vi "peak_value_calculate_A_4_zero_negatives.vi"(0 "IO Module\\AI 1 Data N-1 2":i16, 1 "IO Module\\AI 1 Data N-2 3":i16, 2 "IO Module\\AI 1 Data N-2 2":i16, 3 "Boolean in":bool, 4 "IO Module\\AI 1 Data N-3 2":i16, 6 "IO Module\\AI 1 Data N 3":i16, 7 "IO Module\\AI 1 Data N":i16, 8 "IO Module\\AI 1 Data N-1 3":i16, 9 "IO Module\\AI 1 Data N-3":i16, 10 "IO Module\\AI 1 Data N 2":i16, 11 "IO Module\\AI 1 Data N-1":i16, 13 "IO Module\\AI 1 Data N-2":i16) -> (15 "Read Ready":bool, 16 "Spike Value":i16)   [LabVIEW 2017]
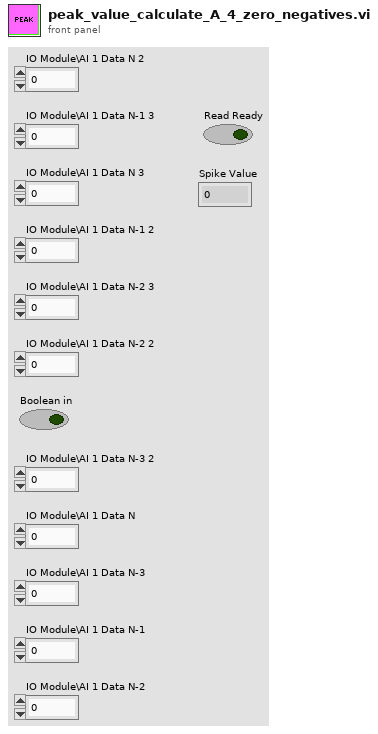
[diagram p1: front panel]
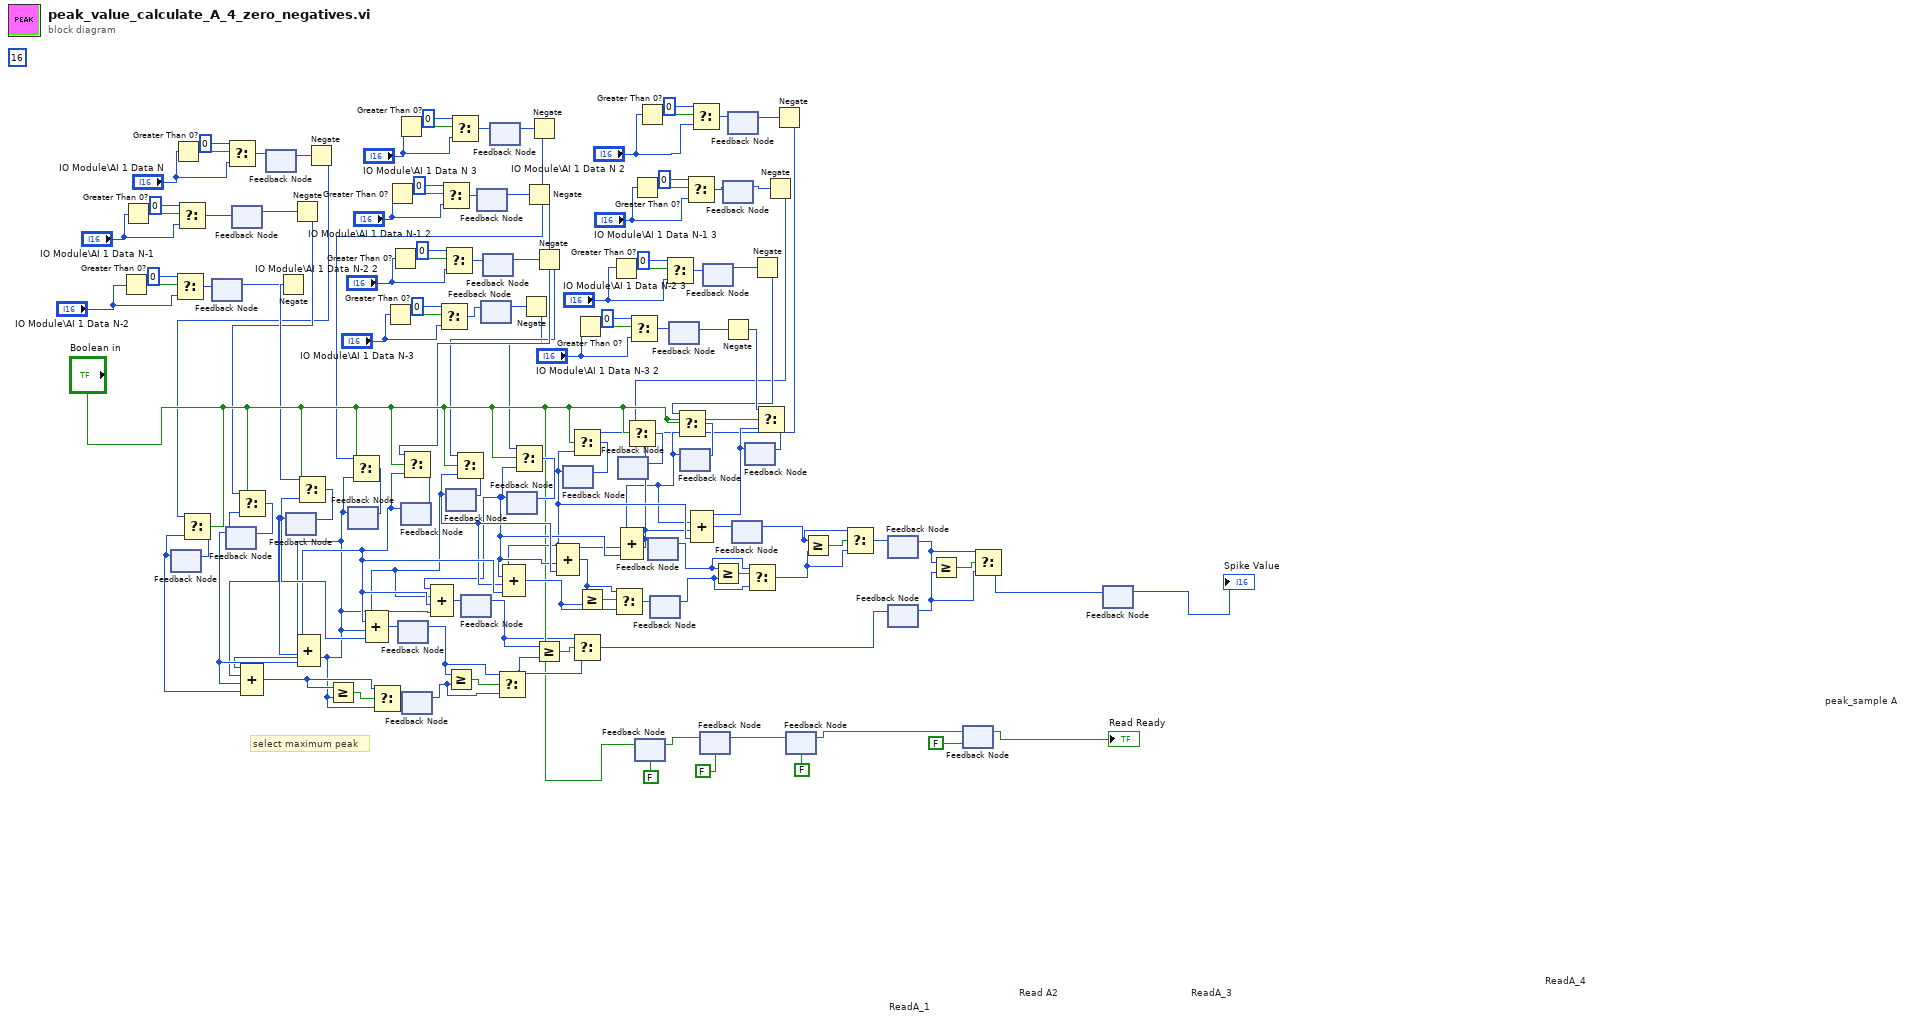
[diagram p0: block diagram]
diagram:
  (unwired) 16
  # "select maximum peak"
  n1 = Greater Than 0?(x="IO Module\\AI 1 Data N-2") -> (x > 0?=w43:bool)
  n2 = Greater Than 0?(x="IO Module\\AI 1 Data N-1") -> (x > 0?=w46:bool)
  n3 = feedback #1() -> (w110:i16)  [unwired: 1 in]
  n4 = Greater Than 0?(x="IO Module\\AI 1 Data N") -> (x > 0?=w49:bool)
  n5 = Select(t=i16 0, s=w43, f="IO Module\\AI 1 Data N-2") -> (s? t:f=w41:i16)
  n6 = Select(t=i16 0, s=w46, f="IO Module\\AI 1 Data N-1") -> (s? t:f=w44:i16)
  n7 = feedback-in #2(w41) -> ()
  n8 = feedback #2() -> (w9:i16)  [unwired: 1 in]
  n9 = feedback #3() -> (w109:i16)  [unwired: 1 in]
  n10 = Select(t=i16 0, s=w49, f="IO Module\\AI 1 Data N") -> (s? t:f=w47:i16)
  n11 = feedback-in #4(w44) -> ()
  n12 = feedback #4() -> (w10:i16)  [unwired: 1 in]
  n13 = feedback-in #5(w47) -> ()
  n14 = feedback #5() -> (w11:i16)  [unwired: 1 in]
  n15 = Negate(x=w9) -> (-x=w22:i16)
  n16 = feedback #6() -> (w106:i16)  [unwired: 1 in]
  n17 = Negate(x=w10) -> (-x=w21:i16)
  n18 = Select(t=w21, s="Boolean in", f=w109) -> (s? t:f=w114:i16)
  n19 = feedback-in #3(w114) -> ()
  n20 = Select(t=w22, s="Boolean in", f=w106) -> (s? t:f=w115:i16)
  n21 = feedback-in #6(w115) -> ()
  n22 = Negate(x=w11) -> (-x=w20:i16)
  n23 = Select(t=w20, s="Boolean in", f=w110) -> (s? t:f=w120:i16)
  n24 = feedback-in #1(w120) -> ()
  n25 = feedback #7() -> (w96:i16)  [unwired: 1 in]
  n26 = Compound Arithmetic op=ADD(w96, w106, w109, w110) -> (w97:i16)
  n27 = Greater Or Equal?(x=w97, y=w96) -> (x >= y?=w98:bool)
  n28 = Select(t=w97, s=w98, f=w96) -> (s? t:f=w122:i16)
  n29 = Greater Than 0?(x="IO Module\\AI 1 Data N-3") -> (x > 0?=w52:bool)
  n30 = Greater Than 0?(x="IO Module\\AI 1 Data N-1 2") -> (x > 0?=w58:bool)
  n31 = Greater Than 0?(x="IO Module\\AI 1 Data N-2 2") -> (x > 0?=w55:bool)
  n32 = Greater Than 0?(x="IO Module\\AI 1 Data N 3") -> (x > 0?=w61:bool)
  n33 = feedback #8() -> (w18:i16)  [unwired: 1 in]
  n34 = feedback #9() -> (w105:i16)  [unwired: 1 in]
  n35 = Compound Arithmetic op=ADD(w105, w96, w106, w109) -> ()  [unwired: 1 out]
  n36 = feedback-in #10(w122) -> ()
  n37 = feedback #10() -> (w19:i16)  [unwired: 1 in]
  n38 = Select(t=i16 0, s=w52, f="IO Module\\AI 1 Data N-3") -> (s? t:f=w50:i16)
  n39 = Select(t=i16 0, s=w58, f="IO Module\\AI 1 Data N-1 2") -> (s? t:f=w56:i16)
  n40 = Select(t=i16 0, s=w55, f="IO Module\\AI 1 Data N-2 2") -> (s? t:f=w53:i16)
  n41 = feedback #11() -> (w104:i16)  [unwired: 1 in]
  n42 = Compound Arithmetic op=ADD(w104, w105, w96, w106) -> (w95:i16)
  n43 = feedback-in #8(w95) -> ()
  n44 = Greater Or Equal?(x=w18, y=w19) -> (x >= y?=w123:bool)
  n45 = Select(t=i16 0, s=w61, f="IO Module\\AI 1 Data N 3") -> (s? t:f=w59:i16)
  n46 = feedback #12() -> (w17:i16)  [unwired: 1 in]
  n47 = feedback-in #13(w56) -> ()
  n48 = feedback #13() -> (w7:i16)  [unwired: 1 in]
  n49 = feedback-in #14(w50) -> ()
  n50 = feedback #14() -> (w5:i16)  [unwired: 1 in]
  n51 = feedback-in #15(w53) -> ()
  n52 = feedback #15() -> (w6:i16)  [unwired: 1 in]
  n53 = feedback-in #16(w59) -> ()
  n54 = feedback #16() -> (w8:i16)  [unwired: 1 in]
  n55 = Select(t=w18, s=w123, f=w19) -> (s? t:f=w92:i16)
  n56 = feedback #17() -> (w103:i16)  [unwired: 1 in]
  n57 = Compound Arithmetic op=ADD(w103, w104, w105, w96) -> (w93:i16)
  n58 = feedback-in #12(w93) -> ()
  n59 = Negate(x=w5) -> (-x=w23:i16)
  n60 = Select(t=w23, s="Boolean in", f=w103) -> (s? t:f=w119:i16)
  n61 = feedback-in #17(w119) -> ()
  n62 = Negate(x=w7) -> (-x=w25:i16)
  n63 = Select(t=w25, s="Boolean in", f=w105) -> (s? t:f=w117:i16)
  n64 = feedback-in #9(w117) -> ()
  n65 = Negate(x=w8) -> (-x=w26:i16)
  n66 = Select(t=w26, s="Boolean in", f=w96) -> (s? t:f=w121:i16)
  n67 = feedback-in #7(w121) -> ()
  n68 = Negate(x=w6) -> (-x=w24:i16)
  n69 = Select(t=w24, s="Boolean in", f=w104) -> (s? t:f=w118:i16)
  n70 = feedback-in #11(w118) -> ()
  n71 = Greater Or Equal?(x=w17, y=w92) -> (x >= y?=w94:bool)
  n72 = feedback #18() -> (w102:i16)  [unwired: 1 in]
  n73 = Compound Arithmetic op=ADD(w102, w103, w104, w105) -> (w90:i16)
  n74 = Select(t=w17, s=w94, f=w92) -> (s? t:f=w91:i16)
  n75 = Greater Than 0?(x="IO Module\\AI 1 Data N-3 2") -> (x > 0?=w64:bool)
  n76 = Greater Than 0?(x="IO Module\\AI 1 Data N-2 3") -> (x > 0?=w67:bool)
  n77 = feedback #19() -> (w101:i16)  [unwired: 1 in]
  n78 = Compound Arithmetic op=ADD(w101, w102, w103, w104) -> (w89:i16)
  n79 = Greater Or Equal?(x=w89, y=w90) -> (x >= y?=w124:bool)
  n80 = Select(t=w89, s=w124, f=w90) -> (s? t:f=w125:i16)
  n81 = Select(t=i16 0, s=w64, f="IO Module\\AI 1 Data N-3 2") -> (s? t:f=w62:i16)
  n82 = Greater Than 0?(x="IO Module\\AI 1 Data N-1 3") -> (x > 0?=w70:bool)
  n83 = feedback #20 "ReadA_1"(FALSE ("Boolean in")) -> (w75:bool)
  n84 = feedback-in #20("Boolean in") -> ()
  n85 = Greater Than 0?(x="IO Module\\AI 1 Data N 2") -> (x > 0?=w74:bool)
  n86 = feedback #21() -> (w15:i16)  [unwired: 1 in]
  n87 = feedback-in #22(w125) -> ()
  n88 = feedback #22() -> (w16:i16)  [unwired: 1 in]
  n89 = Select(t=i16 0, s=w67, f="IO Module\\AI 1 Data N-2 3") -> (s? t:f=w65:i16)
  n90 = feedback-in #23(w62) -> ()
  n91 = feedback #23() -> (w1:i16)  [unwired: 1 in]
  n92 = feedback #24() -> (w100:i16)  [unwired: 1 in]
  n93 = Compound Arithmetic op=ADD(w100, w101, w101, w103) -> (w88:i16)
  n94 = feedback-in #21(w88) -> ()
  n95 = Select(t=i16 0, s=w70, f="IO Module\\AI 1 Data N-1 3") -> (s? t:f=w68:i16)
  n96 = Select(t=i16 0, s=w74, f="IO Module\\AI 1 Data N 2") -> (s? t:f=w71:i16)
  n97 = feedback-in #25(w75) -> ()
  n98 = feedback #25 "Read A2"(FALSE ("Boolean in")) -> (w13:bool)
  n99 = feedback-in #26(w65) -> ()
  n100 = feedback #26() -> (w2:i16)  [unwired: 1 in]
  n101 = Greater Or Equal?(x=w15, y=w16) -> (x >= y?=w126:bool)
  n102 = feedback-in #27(w68) -> ()
  n103 = feedback #27() -> (w3:i16)  [unwired: 1 in]
  n104 = Negate(x=w1) -> (-x=w30:i16)
  n105 = feedback-in #28(w71) -> ()
  n106 = feedback #28() -> (w4:i16)  [unwired: 1 in]
  n107 = feedback #29() -> (w14:i16)  [unwired: 1 in]
  n108 = feedback #30() -> (w99:i16)  [unwired: 1 in]
  n109 = Compound Arithmetic op=ADD(w99, w100, w101, w102) -> (w86:i16)
  n110 = feedback-in #29(w86) -> ()
  n111 = Select(t=w15, s=w126, f=w16) -> (s? t:f=w85:i16)
  n112 = Negate(x=w2) -> (-x=w29:i16)
  n113 = Select(t=w29, s="Boolean in", f=w100) -> (s? t:f=w111:i16)
  n114 = feedback-in #24(w111) -> ()
  n115 = Select(t=w30, s="Boolean in", f=w99) -> (s? t:f=w116:i16)
  n116 = feedback-in #30(w116) -> ()
  n117 = Negate(x=w3) -> (-x=w28:i16)
  n118 = Select(t=w28, s="Boolean in", f=w101) -> (s? t:f=w112:i16)
  n119 = feedback-in #19(w112) -> ()
  n120 = Negate(x=w4) -> (-x=w27:i16)
  n121 = Select(t=w27, s="Boolean in", f=w102) -> (s? t:f=w113:i16)
  n122 = feedback-in #18(w113) -> ()
  n123 = feedback #31 "ReadA_3"(FALSE ("Boolean in")) -> (w127:bool)
  n124 = feedback-in #31(w13) -> ()
  n125 = Greater Or Equal?(x=w14, y=w85) -> (x >= y?=w87:bool)
  n126 = Select(t=w14, s=w87, f=w85) -> (s? t:f=w84:i16)
  n127 = feedback #32() -> (w82:i16)  [unwired: 1 in]
  n128 = feedback-in #32(w84) -> ()
  n129 = feedback #33() -> (w81:i16)  [unwired: 1 in]
  n130 = feedback-in #33(w91) -> ()
  n131 = Greater Or Equal?(x=w82, y=w81) -> (x >= y?=w83:bool)
  n132 = feedback #34 "ReadA_4"(FALSE ("Boolean in")) -> (→"Read Ready":bool)
  n133 = feedback-in #34(w127) -> ()
  n134 = Select(t=w82, s=w83, f=w81) -> (s? t:f=w78:i16)
  n135 = feedback #35 "peak_sample A"() -> (→"Spike Value":i16)  [unwired: 1 in]
  n136 = feedback-in #35(w78) -> ()
